vi "Test Namer With Shared Approved Path default behavior.vi"   [LabVIEW 2020, in "Namer.Tests.lvclass"]
uses:
  Namer.Tests.lvclass
  Source/Approval Tests/Namer With Shared Approved File/Namer With Shared Approved File.lvclass
  Source/Approval Tests/Naming Data/Naming Data.lvclass
  Source/Approval Tests/Naming Data/Naming Data.lvclass/Naming Data.ctl
  Namer.Tests.lvclass/Namer.Tests.ctl
  <vilib>/addons/_JKI Toolkits/Caraya/classes/Test/Test.lvclass
  <vilib>/addons/_JKI Toolkits/Caraya/classes/Assert/Assert.lvclass
  <vilib>/addons/_JKI Toolkits/Caraya/classes/Assert/Assert Equal Value and Type_Variant.vi
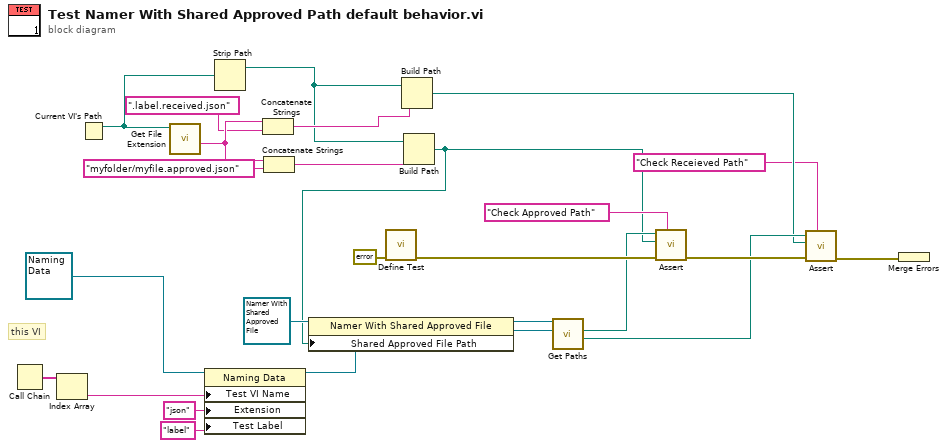
[diagram p0: block diagram]
diagram:
  # "this VI"
  n1 = Call Chain() -> (call chain=w20:string[])
  n2 = Index Array(array=w20) -> (element=w19:string)  [unwired: 1 in]
  n3 = Current VI's Path() -> (path=w13:path)
  n4 = call <vilib>:"Get File Extension.vi"("file"=w13) -> ("filename without extension"=w12:string)  [unwired: 6 in, 4 out]
  n5 = property on="Property Node" class="Naming Data"(reference=refnum<class "Naming Data.lvclass"> refnum ("Naming Data"), "Test VI Name"=w19, "Extension"="json", "Test Label"="label") -> (reference out=w18:refnum<class "Naming Data.lvclass">)  [unwired: 1 in, 1 out]
  n6 = Strip Path(path=w13) -> (stripped path=w3:path)  [unwired: 1 out]
  n7 = Concatenate Strings(w12, ".label.received.json" ("string")) -> (w9:string)
  n8 = Concatenate Strings(w12, "myfolder/myfile.approved.json" ("string")) -> (w8:string)
  n9 = call <vilib>:"Define Test.vi"("error in (no error)"=errorcluster {"status"=FALSE, "code"=0, "source"=""}) -> ("error out"=w24:errorcluster)  [unwired: 9 in, 1 out]
  n10 = Build Path(base path=w3, name or relative path=w9) -> (appended path=w7:path)
  n11 = Build Path(base path=w3, name or relative path=w8) -> (appended path=w1:path)
  n12 = property class="Namer With Shared Approved File"(reference=refnum<class "Namer With Shared Approved File.lvclass"> refnum ("Approval Tests:Namer with SubFolder.lvclass"), "Shared Approved File Path"=w1) -> (reference out=w2:refnum<class "Namer With Shared Approved File.lvclass">)  [unwired: 1 in, 1 out]
  n13 = call-dynamic "Get Paths.vi"("Naming Data"=w18, "Namer With Shared Approved File in"=w2) -> ("Received Path"=w14:path, "Approved Path"=w15:path)  [unwired: 6 in, 2 out]
  n14 = call-poly <vilib>:"Assert.vi"("Label"="Check Approved Path" ("Label (VI Title)"), "error in (no error)"=w24, "Actual"=w1, "Expected"=w15) -> ("error out"=w17:errorcluster)  [unwired: 6 in, 1 out]
  n15 = call-poly <vilib>:"Assert.vi"("Label"="Check Receieved Path" ("Label (VI Title)"), "error in (no error)"=w17, "Actual"=w7, "Expected"=w14) -> ("error out"=w16:errorcluster)  [unwired: 6 in, 1 out]
  n16 = Merge Errors(w16) -> ()  [unwired: 1 out]
